vi "c_GENERATE_OPERATIONS.vi"(11 "FiringOrder":refnum<vi>[](array[refnum])) -> (3 "Array":refnum<class "CodeElement.lvclass">[](array[class]))   [LabVIEW 2017]
uses:
  CodeElements/Base/CodeElement.lvclass
  CodeElements/RawCodeElement_class/RawCodeElement.lvclass
  E:/Code_Generator/CodeElements/Base/CodeElement.lvclass
  CodeElements/Typedef_Element_class/Typedef_Element.lvclass
  CodeElements/SwitchCaseElement_class/SwitchCaseElement.lvclass
  CodeElements/SetIntermediateValueDoLast_class/SetIntermediateValueDoLast.lvclass
  CodeElements/SetIntermediateValue_class/SetIntermediateValue.lvclass
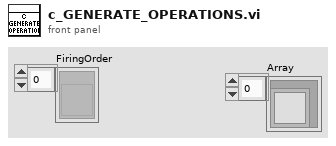
[diagram p1: front panel]
types:
  T1 = cluster{"Array":refnum<class "CodeElement.lvclass">[]}
  T2 = cluster{"CodeElements":refnum<class "CodeElement.lvclass">[]}
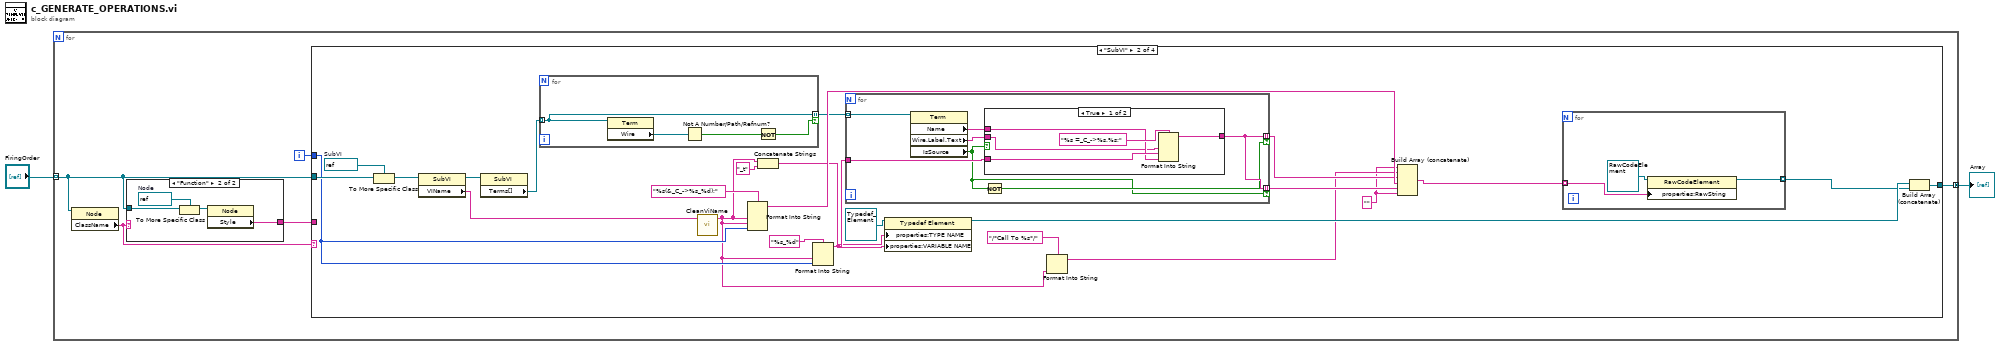
[diagram p0: block diagram]
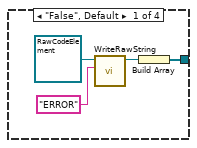
[diagram p2: hidden frame]
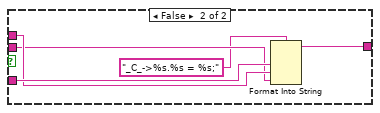
[diagram p3: hidden frame]
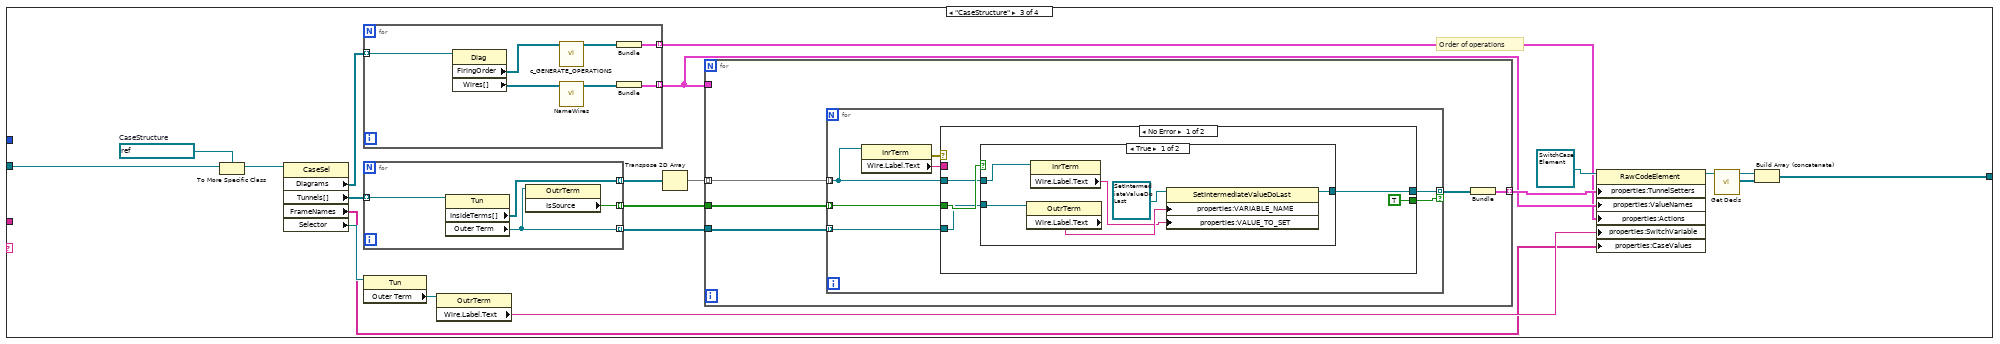
[diagram p4: hidden frame]
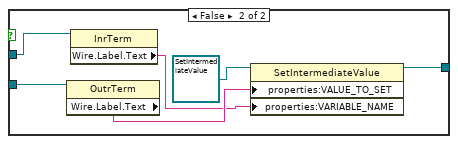
[diagram p5: hidden frame]
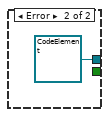
[diagram p6: hidden frame]
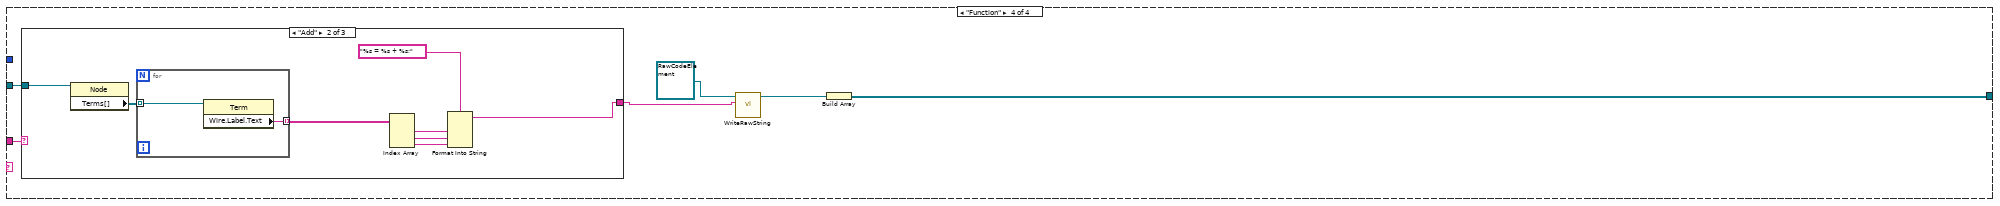
[diagram p7: hidden frame]
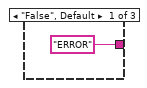
[diagram p8: hidden frame]
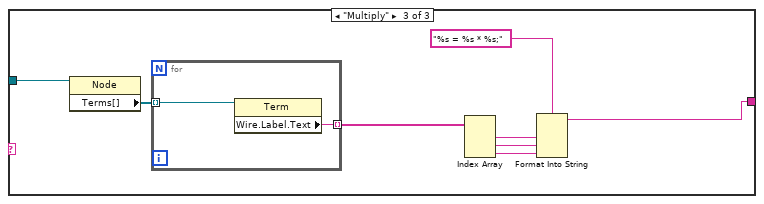
[diagram p9: hidden frame]
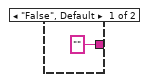
[diagram p10: hidden frame]
diagram:
  n1 = for {
    tunnel: "FiringOrder" -> [w5] mode=indexing
    tunnel: [w4] -> w1 mode=concatenating
    i -> [w3]
    n2 = property class="Node"(reference=w5) -> ("ClassName"=w7:string)  [unwired: 1 in, 2 out]
    n3 = case shown="\"Function\"" w7 {
      tunnel: w5 -> [_ w154]
      tunnel: ["" ("Desc") w151] -> w6
      frame "False", Default {
      }
      frame "Function" {
        w153 = refnum<vi> refnum  # Node
        n4 = To More Specific Class(target class=w153, reference=w154) -> (specific class reference=w152:refnum<vi>)  [unwired: 1 in, 1 out]
        n5 = property class="Node"(reference=w152) -> ("Style"=w151:string)  [unwired: 1 in, 2 out]
      }
    }
    n6 = case shown="\"SubVI\"" w7 {
      tunnel: w6 -> [_ _ _ w128]
      tunnel: w5 -> [_ w36 w81 w127]
      tunnel: [w9 w19 w70 w123] -> w4
      tunnel: w3 -> [_ w29 _ _]
      frame "False", Default {
        n7 = call-dynamic "WriteRawString.vi"("RawString"="ERROR", "object in"=refnum<class "RawCodeElement.lvclass"> refnum) -> ("object out"=w10:refnum<class "RawCodeElement.lvclass">)  [unwired: 8 in, 1 out]
        n8 = Build Array(w10) -> (w9:refnum<class "RawCodeElement.lvclass">[])
      }
      frame "SubVI" {
        w12 = ""
        w35 = refnum<vi> refnum  # SubVI
        n9 = To More Specific Class(target class=w35, reference=w36) -> (specific class reference=w34:refnum<vi>)  [unwired: 1 in, 1 out]
        n10 = property class="SubVI"(reference=w34) -> (reference out=w28:refnum<vi>, "VIName"=w33:string)  [unwired: 1 in, 1 out]
        n11 = property class="SubVI"(reference=w28) -> ("Terms[]"=w25:refnum<vi>[])  [unwired: 1 in, 2 out]
        n12 = for {
          tunnel: w25 -> [w43] mode=indexing
          tunnel: [w43] -> w24 mode=indexing if=w40
          n13 = property class="Term"(reference=w43) -> ("Wire"=w42:refnum<vi>)  [unwired: 1 in, 2 out]
          n14 = Not A Number/Path/Refnum?(number/path/refnum=w42) -> (NaN/Path/Refnum?=w41:bool)
          n15 = Not(x=w41) -> (.not. x?=w40:bool)
        }
        n16 = call "CleanViName.vi"("Name"=w33) -> ("submatch 1"=w14:string)  [unwired: 10 in]
        n17 = Format Into String(format string="%s(&_C_->%s_%d);", w14, w14, w29) -> (resulting string=w31:string)  [unwired: 2 in, 1 out]
        n18 = Concatenate Strings(w14, "_t" ("string")) -> (w18:string)
        n19 = Format Into String(format string="%s_%d", w14, w29) -> (resulting string=w22:string)  [unwired: 2 in, 1 out]
        n20 = for {
          tunnel: w24 -> [w50] mode=indexing
          tunnel: w22 -> [w49]
          tunnel: [w46] -> w27 mode=indexing if=w45
          tunnel: [w46] -> w26 mode=indexing if=w44
          n21 = property class="Term"(reference=w50) -> ("Name"=w48:string, "Wire.Label.Text"=w47:string, "IsSource"=w44:bool)  [unwired: 1 in, 2 out]
          n22 = Not(x=w44) -> (.not. x?=w45:bool)
          n23 = case shown="True" w44 {
            tunnel: w49 -> [w53 w60]
            tunnel: w48 -> [w52 w59]
            tunnel: w47 -> [w51 w58]
            tunnel: [w55 w57] -> w46
            frame True {
              n24 = Format Into String(format string="%s =_C_->%s.%s;", w51, w53, w52) -> (resulting string=w55:string)  [unwired: 2 in, 1 out]
            }
            frame False {
              n25 = Format Into String(format string="_C_->%s.%s = %s;", w60, w59, w58) -> (resulting string=w57:string)  [unwired: 2 in, 1 out]
            }
          }
        }
        n26 = property class="Typedef Element"(reference=refnum<class "Typedef_Element.lvclass"> refnum ("Typedef Element"), "properties:TYPE NAME"=w18, "properties:VARIABLE NAME"=w22) -> (reference out=w21:refnum<class "Typedef_Element.lvclass">)  [unwired: 1 in, 1 out]
        n27 = Format Into String(format string="/*Call To %s*/", w14) -> (resulting string=w13:string)  [unwired: 2 in, 1 out]
        n28 = Build Array (concatenate)(w12, w13, w27, w31, w26, w12) -> (w16:string[])
        n29 = for {
          tunnel: [w39] -> w20 mode=indexing
          tunnel: w16 -> [w37] mode=indexing
          n30 = property class="RawCodeElement"(reference=refnum<class "RawCodeElement.lvclass"> refnum ("RawCodeElement.lvclass"), "properties:RawString"=w37) -> (reference out=w39:refnum<class "RawCodeElement.lvclass">)  [unwired: 1 in, 1 out]
        }
        n31 = Build Array (concatenate)(w21, w20) -> (w19:refnum<class "CodeElement.lvclass">[])
      }
      frame "CaseStructure" {
        w80 = refnum<vi> refnum  # CaseStructure
        # "Order of operations"
        n32 = To More Specific Class(target class=w80, reference=w81) -> (specific class reference=w79:refnum<vi>)  [unwired: 1 in, 1 out]
        n33 = property class="CaseSel"(reference=w79) -> ("Diagrams"=w78:refnum<vi>[], "Tunnels[]"=w68:refnum<vi>[], "FrameNames"=w69:string[], "Selector"=w77:refnum<vi>)  [unwired: 1 in, 2 out]
        n34 = for {
          tunnel: w78 -> [w122] mode=indexing
          tunnel: [w118] -> w73 mode=indexing
          tunnel: [w116] -> w72 mode=indexing
          n35 = property class="Diag"(reference=w122) -> ("FiringOrder"=w121:refnum<vi>[], "Wires[]"=w120:refnum<vi>[])  [unwired: 1 in, 2 out]
          n36 = call "c_GENERATE_OPERATIONS.vi"("FiringOrder"=w121) -> ("Array"=w117:refnum<class "CodeElement.lvclass">[])  [unwired: 10 in]
          n37 = call "NameWires.vi"("Wires[]"=w120) -> ("CodeElements"=w119:refnum<class "CodeElement.lvclass">[])  [unwired: 10 in]
          n38 = Bundle("Array"=w117) -> (w116:T1)  [unwired: 1 in]
          n39 = Bundle("CodeElements"=w119) -> (w118:T2)  [unwired: 1 in]
        }
        n40 = for {
          tunnel: w68 -> [w85] mode=indexing
          tunnel: [w84] -> w67 mode=indexing
          tunnel: [w83] -> w65 mode=indexing
          tunnel: [w82] -> w64 mode=indexing
          n41 = property class="Tun"(reference=w85) -> ("InsideTerms[]"=w84:refnum<vi>[], "Outer Term"=w83:refnum<vi>)  [unwired: 1 in, 2 out]
          n42 = property class="OutrTerm"(reference=w83) -> ("IsSource"=w82:bool)  [unwired: 1 in, 2 out]
        }
        n43 = property class="Tun"(reference=w77) -> ("Outer Term"=w76:refnum<vi>)  [unwired: 1 in, 2 out]
        n44 = property class="OutrTerm"(reference=w76) -> ("Wire.Label.Text"=w71:string)  [unwired: 1 in, 2 out]
        n45 = Transpose 2D Array(2D array=w67) -> (transposed array=w66:refnum<vi>[][])
        n46 = for {
          tunnel: [w90] -> w74 mode=indexing
          tunnel: w73 -> [_]
          tunnel: w66 -> [w88] mode=indexing
          tunnel: w65 -> [w87]
          tunnel: w64 -> [w89]
          n47 = for {
            tunnel: w89 -> [w97] mode=indexing
            tunnel: w87 -> [w96] mode=indexing
            tunnel: w88 -> [w93] mode=indexing
            tunnel: [w95] -> w86 mode=indexing if=w94
            n48 = property class="InrTerm"(reference=w93) -> (error out=w92:errorcluster, "Wire.Label.Text"=w91:string)  [unwired: 1 in, 1 out]
            n49 = case shown="No Error" w92 {
              tunnel: w97 -> [w102 _]
              tunnel: w96 -> [w101 _]
              tunnel: [w100 refnum<class "CodeElement.lvclass"> refnum ("SetReturnValue")] -> w95
              tunnel: w93 -> [w99 _]
              tunnel: [TRUE _] -> w94
              tunnel: w91 -> [_ _]
              frame No Error {
                n50 = case shown="True" w102 {
                  tunnel: w101 -> [w106 w111]
                  tunnel: w99 -> [w107 w110]
                  tunnel: [w105 w113] -> w100
                  frame True {
                    n51 = property class="OutrTerm"(reference=w106) -> ("Wire.Label.Text"=w104:string)  [unwired: 1 in, 2 out]
                    n52 = property class="InrTerm"(reference=w107) -> ("Wire.Label.Text"=w103:string)  [unwired: 1 in, 2 out]
                    n53 = property class="SetIntermediateValueDoLast"(reference=refnum<class "SetIntermediateValueDoLast.lvclass"> refnum ("SetIntermediateValueDoLast"), "properties:VARIABLE_NAME"=w104, "properties:VALUE_TO_SET"=w103) -> (reference out=w105:refnum<class "SetIntermediateValueDoLast.lvclass">)  [unwired: 1 in, 1 out]
                  }
                  frame False {
                    n54 = property class="OutrTerm"(reference=w111) -> ("Wire.Label.Text"=w112:string)  [unwired: 1 in, 2 out]
                    n55 = property class="InrTerm"(reference=w110) -> ("Wire.Label.Text"=w109:string)  [unwired: 1 in, 2 out]
                    n56 = property class="SetIntermediateValue"(reference=refnum<class "SetIntermediateValue.lvclass"> refnum ("SetReturnValue"), "properties:VALUE_TO_SET"=w112, "properties:VARIABLE_NAME"=w109) -> (reference out=w113:refnum<class "SetIntermediateValue.lvclass">)  [unwired: 1 in, 1 out]
                  }
                }
              }
              frame Error {
              }
            }
          }
          n57 = Bundle(w86) -> (w90:cluster{refnum<class "CodeElement.lvclass">[]})  [unwired: 1 in]
        }
        n58 = property class="RawCodeElement"(reference=refnum<class "SwitchCaseElement.lvclass"> refnum ("RawCodeElement"), "properties:TunnelSetters"=w74, "properties:ValueNames"=w73, "properties:Actions"=w72, "properties:SwitchVariable"=w71, "properties:CaseValues"=w69) -> (reference out=w63:refnum<class "SwitchCaseElement.lvclass">)  [unwired: 1 in, 1 out]
        n59 = call-dynamic "Get Decls.vi"("object in"=w63) -> ("Declarations"=w61:refnum<class "CodeElement.lvclass">[], "object out"=w62:refnum<class "SwitchCaseElement.lvclass">)  [unwired: 8 in, 1 out]
        n60 = Build Array (concatenate)(w62, w61) -> (w70:refnum<class "CodeElement.lvclass">[])
      }
      frame "Function" {
        n61 = case shown="\"Add\"" w128 {
          tunnel: w127 -> [_ w137 w147]
          tunnel: ["ERROR" w130 w140] -> w125
          frame "False", Default {
          }
          frame "Add" {
            n62 = property class="Node"(reference=w137) -> ("Terms[]"=w136:refnum<vi>[])  [unwired: 1 in, 2 out]
            n63 = for {
              tunnel: w136 -> [w139] mode=indexing
              tunnel: [w138] -> w135 mode=indexing
              n64 = property class="Term"(reference=w139) -> ("Wire.Label.Text"=w138:string)  [unwired: 1 in, 2 out]
            }
            n65 = Index Array(array=w135) -> (element #1=w133:string, element #2=w132:string, element #3=w131:string)  [unwired: 3 in]
            n66 = Format Into String(format string="%s = %s + %s;", w133, w132, w131) -> (resulting string=w130:string)  [unwired: 2 in, 1 out]
          }
          frame "Multiply" {
            n67 = property class="Node"(reference=w147) -> ("Terms[]"=w146:refnum<vi>[])  [unwired: 1 in, 2 out]
            n68 = for {
              tunnel: w146 -> [w149] mode=indexing
              tunnel: [w148] -> w145 mode=indexing
              n69 = property class="Term"(reference=w149) -> ("Wire.Label.Text"=w148:string)  [unwired: 1 in, 2 out]
            }
            n70 = Index Array(array=w145) -> (element #1=w143:string, element #2=w142:string, element #3=w141:string)  [unwired: 3 in]
            n71 = Format Into String(format string="%s = %s * %s;", w143, w142, w141) -> (resulting string=w140:string)  [unwired: 2 in, 1 out]
          }
        }
        n72 = call-dynamic "WriteRawString.vi"("RawString"=w125, "object in"=refnum<class "RawCodeElement.lvclass"> refnum ("RawCodeElement.lvclass")) -> ("object out"=w124:refnum<class "RawCodeElement.lvclass">)  [unwired: 8 in, 1 out]
        n73 = Build Array(w124) -> (w123:refnum<class "RawCodeElement.lvclass">[])
      }
    }
  }
  "Array" <- w1
